vi "test-transform3d.vi"(8 "error in (no error)":errorcluster) -> (0 "error out":errorcluster, 3 "All PASSED":bool)   [LabVIEW 2019]
uses:
  <vilib>/Rock Robotics/WPI/ThirdParty/JAS_Junk/TrajLib/Matrix_NormF.vi
  <vilib>/Rock Robotics/WPI/ThirdParty/JAS_Junk/TrajLib/Quaternion_New.vi
  <vilib>/Rock Robotics/WPI/ThirdParty/JAS_Junk/TrajLib/Rotation3d_Create_Default.vi
  <vilib>/Rock Robotics/WPI/ThirdParty/JAS_Junk/TrajLib/Pose3d_New_Default.vi
  <vilib>/Rock Robotics/WPI/ThirdParty/JAS_Junk/TrajLib/Transform3d_Create_Pose3dPose3d.vi
  <vilib>/Rock Robotics/WPI/ThirdParty/JAS_Junk/TrajLib/Pose3d_TransformBy.vi
  <vilib>/Rock Robotics/WPI/ThirdParty/JAS_Junk/TrajLib/Pose3d_getTranslation3d.vi
  <vilib>/Rock Robotics/WPI/ThirdParty/JAS_Junk/TrajLib/Translation3d_GetXYZ.vi
  <vilib>/Rock Robotics/WPI/ThirdParty/JAS_Junk/TrajLib/Quaternion_Get_All.vi
  <vilib>/Rock Robotics/WPI/ThirdParty/JAS_Junk/TrajLib/Rotation3d_GetQuaterion.vi
  <vilib>/Rock Robotics/WPI/ThirdParty/JAS_Junk/TrajLib/Rotation3d_UnaryMinus.vi
  <vilib>/Rock Robotics/WPI/ThirdParty/JAS_Junk/TrajLib/Translation3d_RotateBy.vi
  <vilib>/Rock Robotics/WPI/ThirdParty/JAS_Junk/TrajLib/Translation3d_UnaryMinus.vi
  <vilib>/Rock Robotics/WPI/ThirdParty/JAS_Junk/TrajLib/Transform3d_GetTranslation3d.vi
  <vilib>/Rock Robotics/WPI/ThirdParty/JAS_Junk/TrajLib/Transform3d_GetRotation3d.vi
  <vilib>/Analysis/_algsub.llb/Matrix Norm.vi
  <vilib>/Analysis/_algsub.llb/Real Matrix Norm.vi
  <vilib>/Rock Robotics/WPI/ThirdParty/JAS_Junk/TrajLib/Quaternion_New_Default.vi
  <vilib>/Rock Robotics/WPI/ThirdParty/JAS_Junk/TrajLib/Translation3d_Create_Default.vi
  <vilib>/Rock Robotics/WPI/ThirdParty/JAS_Junk/TrajLib/Translation3d_Minus.vi
  <vilib>/Rock Robotics/WPI/ThirdParty/JAS_Junk/TrajLib/Rotation3d_Minus.vi
  <vilib>/Rock Robotics/WPI/ThirdParty/JAS_Junk/TrajLib/Translation3d_Plus.vi
  <vilib>/Rock Robotics/WPI/ThirdParty/JAS_Junk/TrajLib/Rotation3d_Plus.vi
  <vilib>/Rock Robotics/WPI/ThirdParty/JAS_Junk/TrajLib/Rotation3d_Create_Quaternion.vi
  <vilib>/Rock Robotics/WPI/ThirdParty/JAS_Junk/TrajLib/Quaternion_Inverse.vi
  <vilib>/Rock Robotics/WPI/ThirdParty/JAS_Junk/TrajLib/Quaternion_Times.vi
  <vilib>/Rock Robotics/WPI/ThirdParty/JAS_Junk/TrajLib/Rotation3d_RotateBy.vi
  <vilib>/Rock Robotics/WPI/ThirdParty/JAS_Junk/TrajLib/Quaternion_Normalize.vi
  <vilib>/Rock Robotics/WPI/ThirdParty/JAS_Junk/TrajLib/Quaternion_Get_LVQuat.vi
  <vilib>/Rock Robotics/WPI/ThirdParty/JAS_Junk/TrajLib/Quaternion_New_LVQuat.vi
  <vilib>/Rock Robotics/WPI/ThirdParty/JAS_Junk/TrajLib/Quaternion_Equals.vi
  <vilib>/Analysis/Matrix/Numeric/Conversions/Array To Matrix.vi
  <vilib>/Analysis/Matrix/Numeric/Conversions/Array To Matrix - RA.vi
  <vilib>/robotics/Kinematics/Multiply Quaternions.vi
  <vilib>/robotics/Kinematics/Multiply Quaternion by Quaternion.vi
  <vilib>/Rock Robotics/WPI/ThirdParty/JAS_Junk/TrajLib/Trajectory_Library.lvlib
panel:
  # "Transform3d"
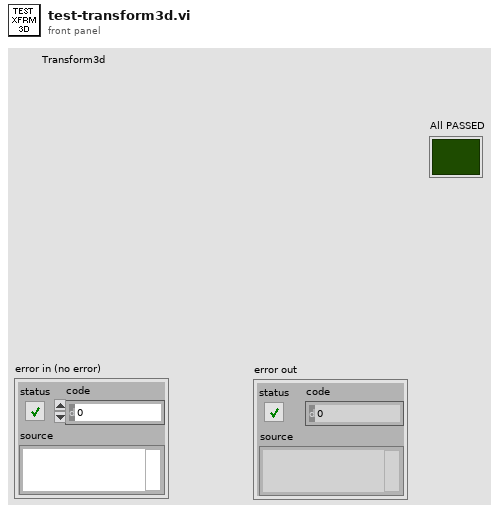
[diagram p1: front panel]
types:
  T1 = typedef "Trajectory_Library.lvlib/TRANSLATION3D.ctl" = cluster{"X":dbl, "Y":dbl, "Z":dbl}
  T2 = typedef "Trajectory_Library.lvlib/ROTATION3D.ctl" = cluster{"Q_quaternion":T3}
  T3 = typedef "Trajectory_Library.lvlib/QUATERNION.ctl" = cluster{"R":dbl, "V":dbl[]}
  T4 = typedef "Trajectory_Library.lvlib/TRANSFORM3D.ctl" = cluster{"TRANSLATION3D":T1, "ROTATION3D":T2}
  T5 = typedef "Trajectory_Library.lvlib/POSE3D.ctl" = cluster{"Translation3d":T1, "Rotation3d":T2}
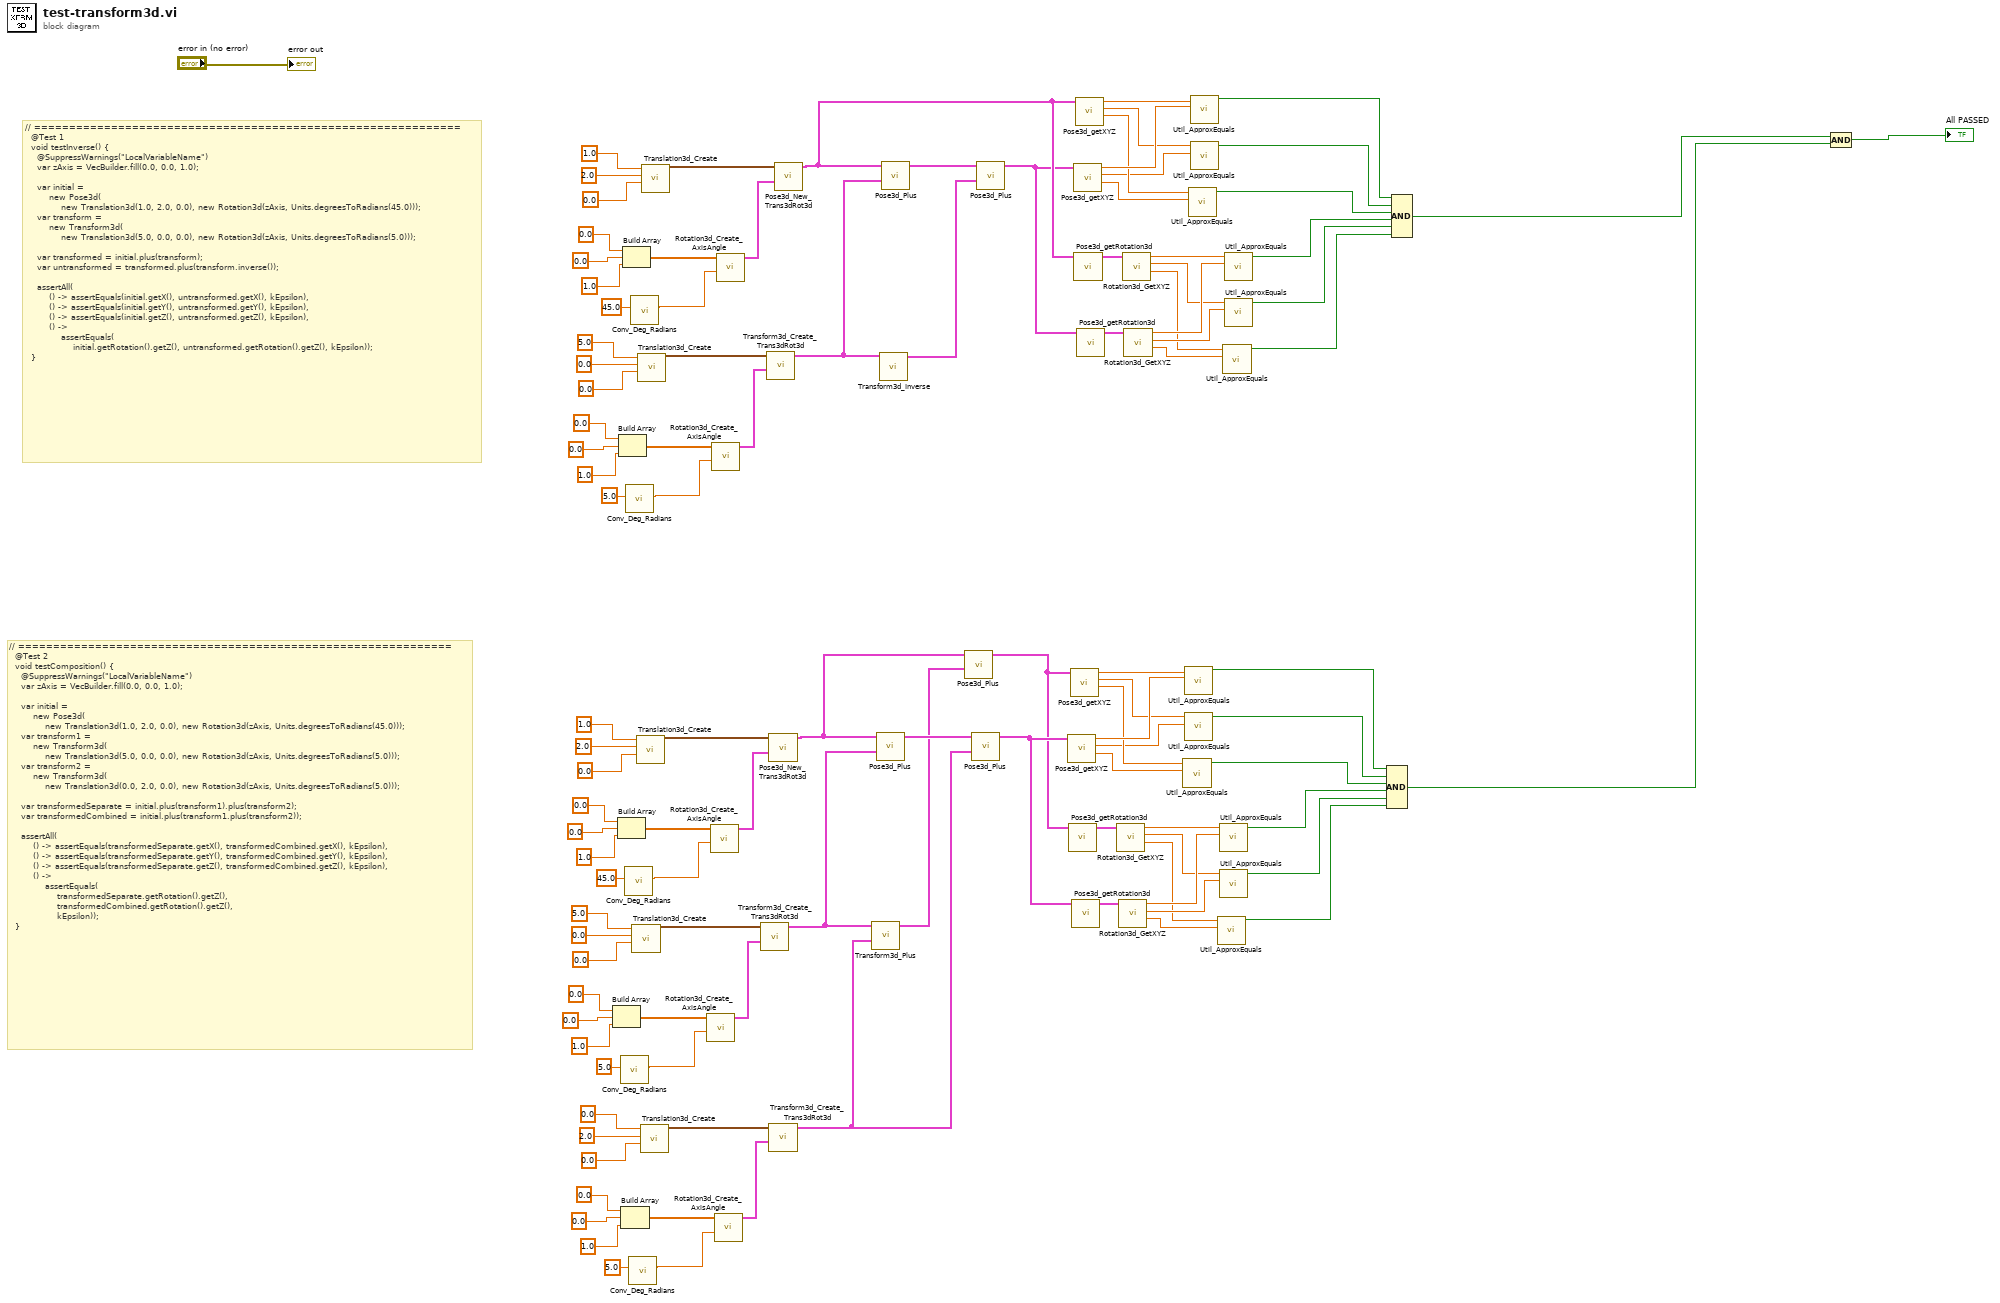
[diagram p0: block diagram]
diagram:
  # "// ==============================================================\n  @Test 2\n  void testComposition() {\n    @SuppressWarnings(\"LocalVariableName\")\n    var zAxis = VecBuilder.fill(0.0, 0.0, 1.0);\n\n    var initial =\n        new Pose3d(\n            new Translation3d(1.0, 2.0, 0.0), new Rotation3d(zAxis, Units.degreesToRadians(45.0)));\n    var transform1 =\n        new Transform3d(\n            new Translation3d(5.0, 0.0, 0.0), new Rotation3d(zAxis, Units.degreesToRadians(5.0)));\n    var transform2 =\n        new Transform3d(\n            new Translation3d(0.0, 2.0, 0.0), new Rotation3d(zAxis, Units.degreesToRadians(5.0)));\n\n    var transformedSeparate = initial.plus(transform1).plus(transform2);\n    var transformedCombined = initial.plus(transform1.plus(transform2));\n\n    assertAll(\n        () -> assertEquals(transformedSeparate.getX(), transformedCombined.getX(), kEpsilon),\n        () -> assertEquals(transformedSeparate.getY(), transformedCombined.getY(), kEpsilon),\n        () -> assertEquals(transformedSeparate.getZ(), transformedCombined.getZ(), kEpsilon),\n        () ->\n            assertEquals(\n                transformedSeparate.getRotation().getZ(),\n                transformedCombined.getRotation().getZ(),\n                kEpsilon));\n  }"
  # "// =============================================================\n  @Test 1\n  void testInverse() {\n    @SuppressWarnings(\"LocalVariableName\")\n    var zAxis = VecBuilder.fill(0.0, 0.0, 1.0);\n\n    var initial =\n        new Pose3d(\n            new Translation3d(1.0, 2.0, 0.0), new Rotation3d(zAxis, Units.degreesToRadians(45.0)));\n    var transform =\n        new Transform3d(\n            new Translation3d(5.0, 0.0, 0.0), new Rotation3d(zAxis, Units.degreesToRadians(5.0)));\n\n    var transformed = initial.plus(transform);\n    var untransformed = transformed.plus(transform.inverse());\n\n    assertAll(\n        () -> assertEquals(initial.getX(), untransformed.getX(), kEpsilon),\n        () -> assertEquals(initial.getY(), untransformed.getY(), kEpsilon),\n        () -> assertEquals(initial.getZ(), untransformed.getZ(), kEpsilon),\n        () ->\n            assertEquals(\n                initial.getRotation().getZ(), untransformed.getRotation().getZ(), kEpsilon));\n  }"
  n1 = Build Array(0.0 ("element"), 0.0 ("element"), 1.0 ("element")) -> (w50:dbl[])
  n2 = Build Array(0.0 ("element"), 0.0 ("element"), 1.0 ("element")) -> (w61:dbl[])
  n3 = Build Array(0.0 ("element"), 0.0 ("element"), 1.0 ("element")) -> (w99:dbl[])
  n4 = call <vilib>:"Conv_Deg_Radians.vi"("Degress"=5.0) -> ("Radians"=w48:dbl)  [unwired: 10 in]
  n5 = Build Array(0.0 ("element"), 0.0 ("element"), 1.0 ("element")) -> (w17:dbl[])
  n6 = Build Array(0.0 ("element"), 0.0 ("element"), 1.0 ("element")) -> (w110:dbl[])
  n7 = call <vilib>:"Conv_Deg_Radians.vi"("Degress"=45.0) -> ("Radians"=w59:dbl)  [unwired: 10 in]
  n8 = call <vilib>:"Conv_Deg_Radians.vi"("Degress"=5.0) -> ("Radians"=w97:dbl)  [unwired: 10 in]
  n9 = call <vilib>:"Conv_Deg_Radians.vi"("Degress"=5.0) -> ("Radians"=w15:dbl)  [unwired: 10 in]
  n10 = call <vilib>:"Conv_Deg_Radians.vi"("Degress"=45.0) -> ("Radians"=w108:dbl)  [unwired: 10 in]
  n11 = call <vilib>:"Translation3d_Create.vi"("Z"=0.0, "Y"=0.0, "X"=5.0) -> ("TRANSLATION3D"=w41:T1)  [unwired: 8 in]
  n12 = call <vilib>:"Translation3d_Create.vi"("Z"=0.0, "Y"=2.0, "X"=1.0) -> ("TRANSLATION3D"=w52:T1)  [unwired: 8 in]
  n13 = call <vilib>:"Translation3d_Create.vi"("Z"=0.0, "Y"=0.0, "X"=5.0) -> ("TRANSLATION3D"=w90:T1)  [unwired: 8 in]
  n14 = call <vilib>:"Translation3d_Create.vi"("Z"=0.0, "Y"=2.0, "X"=0.0) -> ("TRANSLATION3D"=w8:T1)  [unwired: 8 in]
  n15 = call <vilib>:"Translation3d_Create.vi"("Z"=0.0, "Y"=2.0, "X"=1.0) -> ("TRANSLATION3D"=w101:T1)  [unwired: 8 in]
  n16 = call <vilib>:"Rotation3d_Create_AxisAngle.vi"("Angle"=w48, "Axis Vector"=w50) -> ("Rotation3d"=w40:T2)  [unwired: 9 in]
  n17 = call <vilib>:"Rotation3d_Create_AxisAngle.vi"("Angle"=w59, "Axis Vector"=w61) -> ("Rotation3d"=w51:T2)  [unwired: 9 in]
  n18 = call <vilib>:"Rotation3d_Create_AxisAngle.vi"("Angle"=w97, "Axis Vector"=w99) -> ("Rotation3d"=w89:T2)  [unwired: 9 in]
  n19 = call <vilib>:"Rotation3d_Create_AxisAngle.vi"("Angle"=w15, "Axis Vector"=w17) -> ("Rotation3d"=w7:T2)  [unwired: 9 in]
  n20 = call <vilib>:"Rotation3d_Create_AxisAngle.vi"("Angle"=w108, "Axis Vector"=w110) -> ("Rotation3d"=w100:T2)  [unwired: 9 in]
  n21 = call <vilib>:"Transform3d_Create_Trans3dRot3d.vi"("Rotation3d"=w40, "Translation3d"=w41) -> ("Transform3d"=w6:T4)  [unwired: 9 in]
  n22 = call <vilib>:"Transform3d_Create_Trans3dRot3d.vi"("Rotation3d"=w89, "Translation3d"=w90) -> ("Transform3d"=w88:T4)  [unwired: 9 in]
  n23 = call <vilib>:"Pose3d_New_Trans3dRot3d.vi"("Rotation3d"=w51, "Translation3d"=w52) -> ("outPose3d"=w4:T5)  [unwired: 9 in]
  n24 = call <vilib>:"Transform3d_Create_Trans3dRot3d.vi"("Rotation3d"=w7, "Translation3d"=w8) -> ("Transform3d"=w5:T4)  [unwired: 9 in]
  n25 = call <vilib>:"Pose3d_New_Trans3dRot3d.vi"("Rotation3d"=w100, "Translation3d"=w101) -> ("outPose3d"=w85:T5)  [unwired: 9 in]
  n26 = call <vilib>:"Transform3d_Plus.vi"("otherTransform3d"=w5, "in Transform3d"=w6) -> ("Transform3d"=w3:T4)  [unwired: 9 in]
  n27 = call <vilib>:"Pose3d_Plus.vi"("other Transform3d"=w6, "in Pose3d"=w4) -> ("out Pose3d"=w39:T5)  [unwired: 9 in]
  n28 = call <vilib>:"Transform3d_Inverse.vi"("inTransform3d"=w88) -> ("outTransform3d"=w87:T4)  [unwired: 10 in]
  n29 = call <vilib>:"Pose3d_Plus.vi"("other Transform3d"=w88, "in Pose3d"=w85) -> ("out Pose3d"=w86:T5)  [unwired: 9 in]
  n30 = call <vilib>:"Pose3d_Plus.vi"("other Transform3d"=w3, "in Pose3d"=w4) -> ("out Pose3d"=w2:T5)  [unwired: 9 in]
  n31 = call <vilib>:"Pose3d_Plus.vi"("other Transform3d"=w5, "in Pose3d"=w39) -> ("out Pose3d"=w38:T5)  [unwired: 9 in]
  n32 = call <vilib>:"Pose3d_Plus.vi"("other Transform3d"=w87, "in Pose3d"=w86) -> ("out Pose3d"=w84:T5)  [unwired: 9 in]
  n33 = call <vilib>:"Pose3d_getXYZ.vi"("in Pose3d"=w38) -> ("Z"=w32:dbl, "Y"=w33:dbl, "X"=w36:dbl)  [unwired: 8 in]
  n34 = call <vilib>:"Pose3d_getRotation3d.vi"("in Pose3d"=w2) -> ("out Rotation3d"=w31:T2)  [unwired: 10 in]
  n35 = call <vilib>:"Pose3d_getXYZ.vi"("in Pose3d"=w2) -> ("Z"=w34:dbl, "Y"=w35:dbl, "X"=w37:dbl)  [unwired: 8 in]
  n36 = call <vilib>:"Pose3d_getRotation3d.vi"("in Pose3d"=w38) -> ("out Rotation3d"=w30:T2)  [unwired: 10 in]
  n37 = call <vilib>:"Pose3d_getXYZ.vi"("in Pose3d"=w84) -> ("Z"=w78:dbl, "Y"=w79:dbl, "X"=w82:dbl)  [unwired: 8 in]
  n38 = call <vilib>:"Pose3d_getRotation3d.vi"("in Pose3d"=w85) -> ("out Rotation3d"=w77:T2)  [unwired: 10 in]
  n39 = call <vilib>:"Pose3d_getXYZ.vi"("in Pose3d"=w85) -> ("Z"=w80:dbl, "Y"=w81:dbl, "X"=w83:dbl)  [unwired: 8 in]
  n40 = call <vilib>:"Pose3d_getRotation3d.vi"("in Pose3d"=w84) -> ("out Rotation3d"=w76:T2)  [unwired: 10 in]
  n41 = call <vilib>:"Rotation3d_GetXYZ.vi"("in Rotation3d"=w31) -> ("Z"=w25:dbl, "Y"=w27:dbl, "X"=w29:dbl)  [unwired: 8 in]
  n42 = call <vilib>:"Rotation3d_GetXYZ.vi"("in Rotation3d"=w30) -> ("Z"=w24:dbl, "Y"=w26:dbl, "X"=w28:dbl)  [unwired: 8 in]
  n43 = call <vilib>:"Rotation3d_GetXYZ.vi"("in Rotation3d"=w77) -> ("Z"=w71:dbl, "Y"=w73:dbl, "X"=w75:dbl)  [unwired: 8 in]
  n44 = call <vilib>:"Rotation3d_GetXYZ.vi"("in Rotation3d"=w76) -> ("Z"=w70:dbl, "Y"=w72:dbl, "X"=w74:dbl)  [unwired: 8 in]
  n45 = call <vilib>:"Util_ApproxEquals.vi"("Value 2"=w32, "Value 1"=w34) -> ("ApproxEquals"=w21:bool)  [unwired: 9 in]
  n46 = call <vilib>:"Util_ApproxEquals.vi"("Value 2"=w36, "Value 1"=w37) -> ("ApproxEquals"=w23:bool)  [unwired: 9 in]
  n47 = call <vilib>:"Util_ApproxEquals.vi"("Value 2"=w33, "Value 1"=w35) -> ("ApproxEquals"=w22:bool)  [unwired: 9 in]
  n48 = call <vilib>:"Util_ApproxEquals.vi"("Value 2"=w78, "Value 1"=w80) -> ("ApproxEquals"=w67:bool)  [unwired: 9 in]
  n49 = call <vilib>:"Util_ApproxEquals.vi"("Value 2"=w82, "Value 1"=w83) -> ("ApproxEquals"=w69:bool)  [unwired: 9 in]
  n50 = call <vilib>:"Util_ApproxEquals.vi"("Value 2"=w79, "Value 1"=w81) -> ("ApproxEquals"=w68:bool)  [unwired: 9 in]
  n51 = call <vilib>:"Util_ApproxEquals.vi"("Value 2"=w24, "Value 1"=w25) -> ("ApproxEquals"=w18:bool)  [unwired: 9 in]
  n52 = call <vilib>:"Util_ApproxEquals.vi"("Value 2"=w28, "Value 1"=w29) -> ("ApproxEquals"=w20:bool)  [unwired: 9 in]
  n53 = call <vilib>:"Util_ApproxEquals.vi"("Value 2"=w26, "Value 1"=w27) -> ("ApproxEquals"=w19:bool)  [unwired: 9 in]
  n54 = call <vilib>:"Util_ApproxEquals.vi"("Value 2"=w70, "Value 1"=w71) -> ("ApproxEquals"=w64:bool)  [unwired: 9 in]
  n55 = call <vilib>:"Util_ApproxEquals.vi"("Value 2"=w74, "Value 1"=w75) -> ("ApproxEquals"=w66:bool)  [unwired: 9 in]
  n56 = call <vilib>:"Util_ApproxEquals.vi"("Value 2"=w72, "Value 1"=w73) -> ("ApproxEquals"=w65:bool)  [unwired: 9 in]
  n57 = Compound Arithmetic op=AND(w23, w22, w21, w20, w19, w18) -> (w1:bool)
  n58 = Compound Arithmetic op=AND(w69, w68, w67, w66, w65, w64) -> (w62:bool)
  n59 = Compound Arithmetic op=AND(w62, w1) -> (→"All PASSED":bool)
  "error out" <- "error in (no error)"
